vi "Detector_setup.vi"(4 "Samples per channel":i32, 5 "Sample rate (Hz)":dbl, 7 "error in (no error)":errorcluster, 10 "Samp Clk. Delay Units":i32(ring)=10364 items=["Seconds"=10364, "Ticks"=10304], 11 "Sample Clock Delay":dbl, 14 "Sample clock source":tag="/Dev1/PFI0", 17 "Delay from sample clock":bool) -> (20 "task out":refnum<k21>, 27 "error out":errorcluster)   [LabVIEW 2014]
uses:
  <vilib>/DAQmx/create/channels.llb/DAQmx Create Channel (AI-Voltage-Basic).vi
  <vilib>/DAQmx/configure/timing.llb/DAQmx Timing (Sample Clock).vi
  <resource>/objmgr/daqmx.rc
panel:
  in  "Sample Clock Delay 2":dbl
  in  "Z axis":T1
  in  "Slow axis":T1
  in  "Fast axis":T1
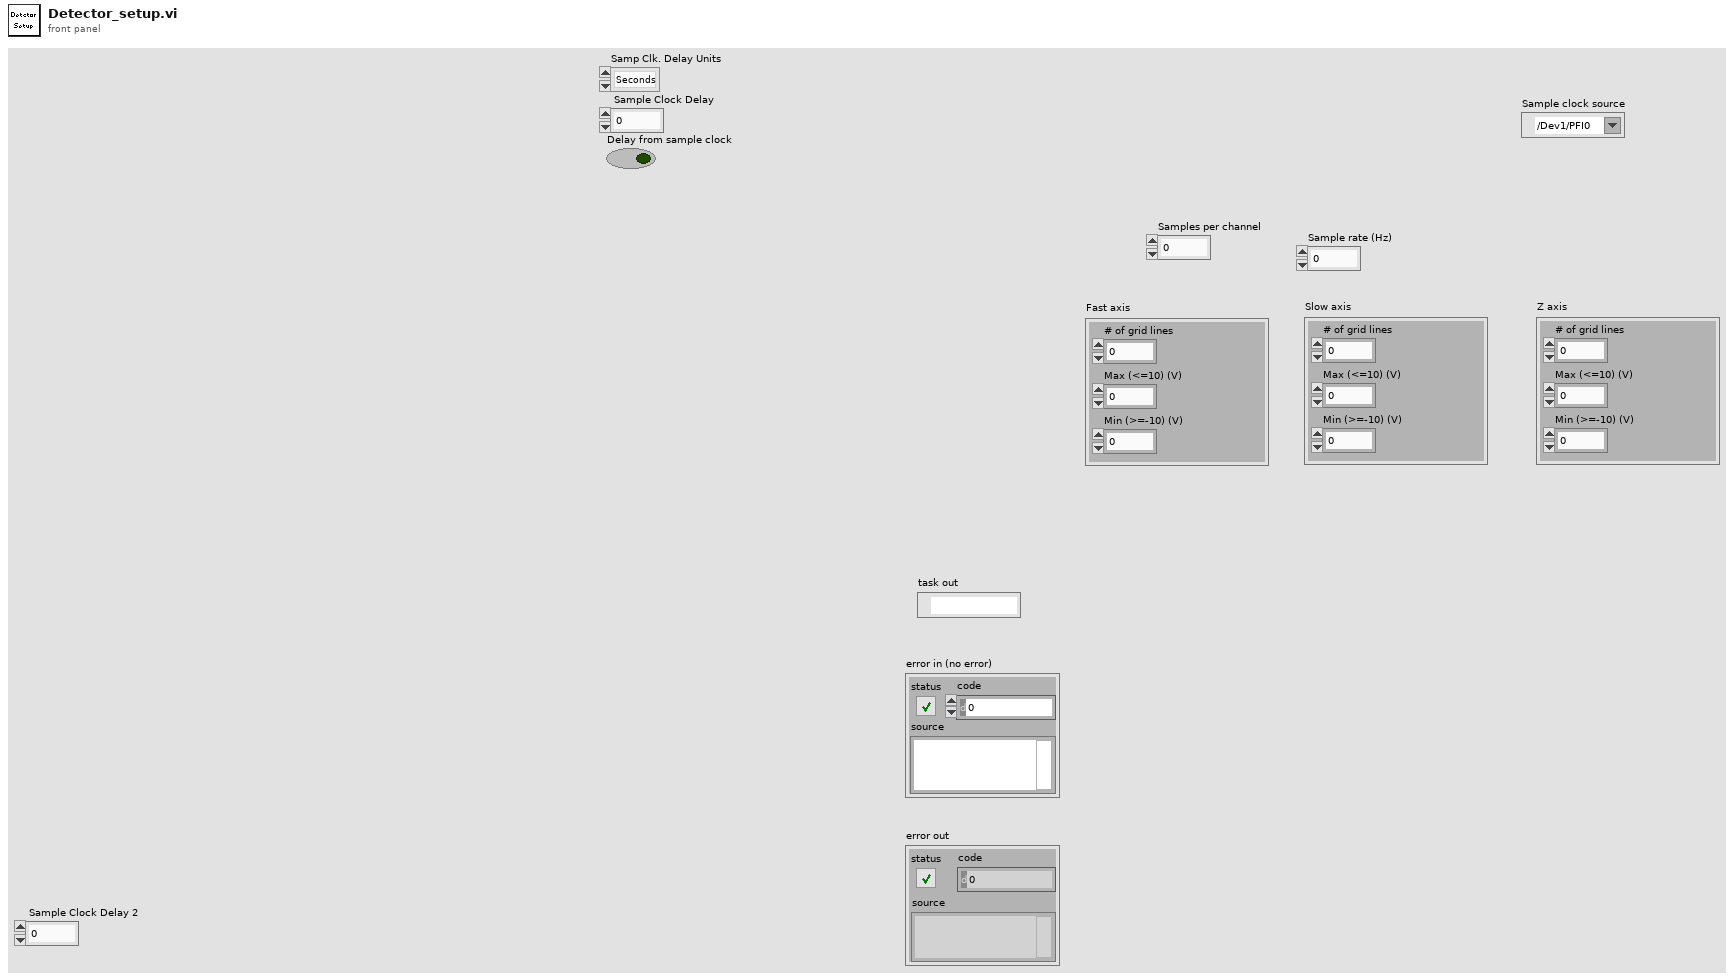
[diagram p1: front panel]
types:
  T1 = cluster{"# of grid lines":u16, "Max (<=10) (V)":dbl, "Min (>=-10) (V)":dbl}
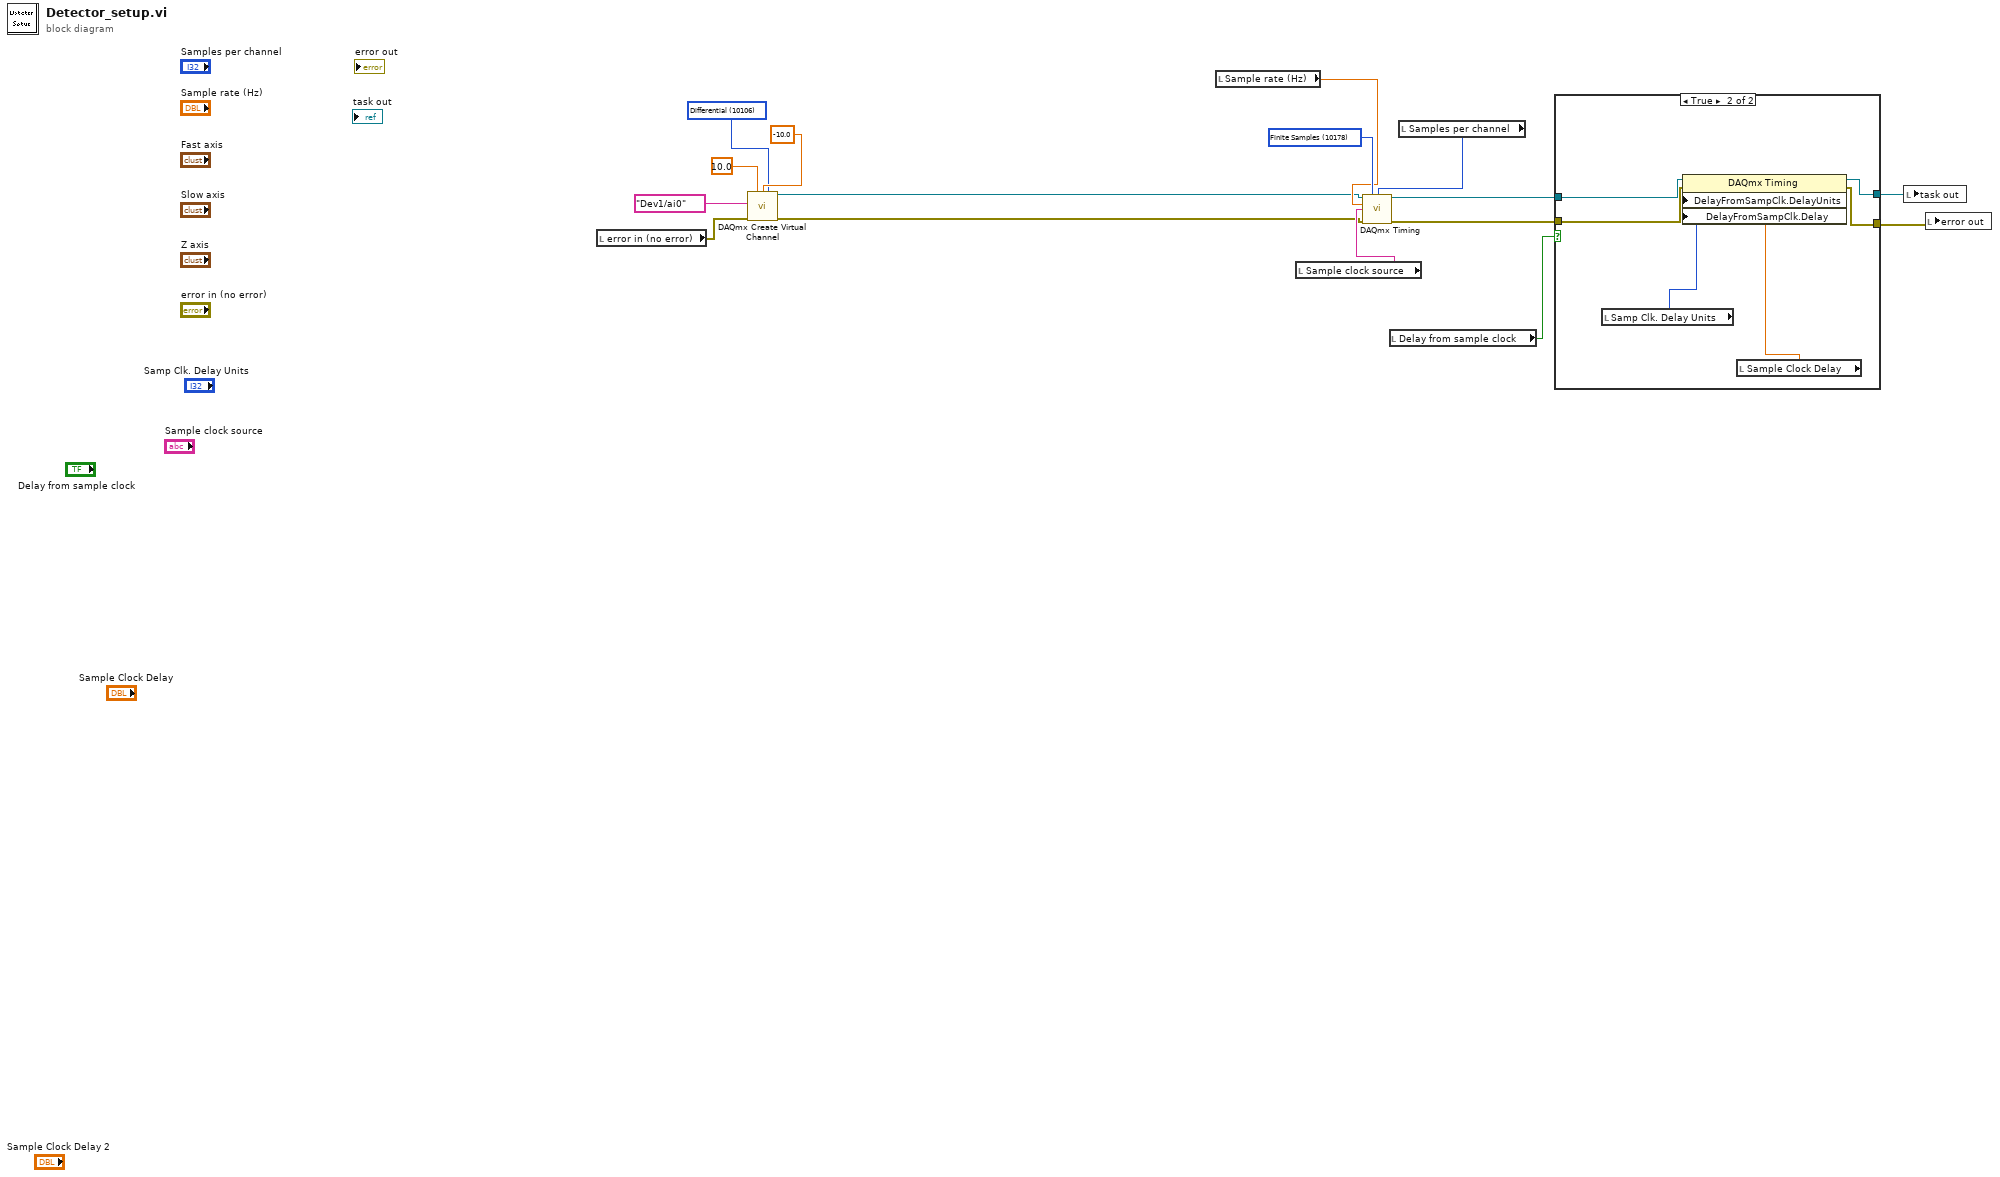
[diagram p0: block diagram]
diagram:
  w13 = 10178 items=["Finite Samples"=10178, "Continuous Samples"=10123, "Hardware Timed Single Point"=12522] ("sample mode")
  w15 = 10106 items=["Default"=-1, "RSE"=10083, "NRSE"=10078, "Differential"=10106, "Pseudodifferential"=12529] ("input terminal configuration")
  n1 = local read "error in (no error)"() -> (w1:errorcluster)
  n2 = call-poly <vilib>:"DAQmx Create Virtual Channel.vi"("maximum value"=10.0, "minimum value"=-10.0, "input terminal configuration"=w15, "physical channels"=tag "Dev1/ai0", "error in"=w1) -> ("task out"=w4:refnum<k21>, "error out"=w3:errorcluster)  [unwired: 9 in]
  n3 = local read "Sample rate (Hz)"() -> (w5:dbl)
  n4 = local read "Sample clock source"() -> (w10:tag)
  n5 = local read "Delay from sample clock"() -> (w2:bool)
  n6 = local read "Samples per channel"() -> (w12:i32)
  n7 = call-poly <vilib>:"DAQmx Timing.vi"("task/channels in"=w4, "sample mode"=w13, "samples per channel"=w12, "rate"=w5, "source"=w10, "error in"=w3) -> ("task out"=w7:refnum<k21>, "error out"=w6:errorcluster)  [unwired: 8 in]
  n8 = case shown="True" w2 {
    tunnel: [w18 w24] -> w9
    tunnel: [w17 w23] -> w8
    tunnel: w7 -> [w18 w22]
    tunnel: w6 -> [w17 w21]
    frame False {
    }
    frame True {
      n9 = local read "Samp Clk. Delay Units"() -> (w19:i32)
      n10 = local read "Sample Clock Delay"() -> (w20:dbl)
      n11 = property class="DAQmx Timing"(reference=w22, error in=w21, "DelayFromSampClk.DelayUnits"=w19, "DelayFromSampClk.Delay"=w20) -> (reference out=w24:refnum<k21>, error out=w23:errorcluster)
    }
  }
  n12 = local write "task out"(w9) -> ()
  n13 = local write "error out"(w8) -> ()
